vi "MagBoard_n64_Serial_Viewer.vi"() -> ()   [LabVIEW 2018]
uses:
  <vilib>/Math Plots/3D Math Plots/3D Surface/3D Surface XCtrl/3D Surface.xctl
  <vilib>/Utility/file.llb/Write Delimited Spreadsheet (DBL).vi
  <vilib>/Utility/file.llb/Read Delimited Spreadsheet (I64).vi
  <vilib>/Math Plots/3D Math Plots/3D Surface/3D Surface Datatype/Public/Plot Helper (Matrix).vi
  <vilib>/Math Plots/3D Math Plots/3D Surface/3D Surface Datatype/3D Surface Datatype.lvclass
panel:
  out "Reading":bool
  out "Initialised":bool
  out "Connected":bool
  in  "Tab Control":T1(tab)
  out "3D Surface":refnum<class "3D Plot Datatype.lvclass">[](xcontrol)
  out "Node XYZ List":dbl[][](array[numeric])
  in  "dT":u32=40
  in  "Axis":enum16{"X", "Y", "Z", "Calib Z"}(ring)
  out "Real dT":u32
  in  "Tare":bool
  out "Initialisation String":string
  out "Data Packet":string
  out "Time":u32=4294745741
  out "Read Count":i32
  out "Sensor Lookup Indices":i32[](array[numeric])
  in  "VISA resource name":refnum<visa-resource-name>="COM7"
  in  "Serial Settings":T2={"baud rate"=115200, "data bits"=8, "parity"=enum."None", "stop bits"=10, "flow control"=0} {"flow control" items=["None"=0, "XON/XOFF"=1, "RTS/CTS"=2, "DTR/DSR"=4]; "stop bits" items=["1.0"=10, "1.5"=15, "2.0"=20]; "data bits" min=5 max=8 step=1; "baud rate" items=["75"=75, "110"=110, "134"=134, "150"=150, "300"=300, "600"=600, "1200"=1200, "1800"=1800, "2400"=2400, "4800"=4800, "7200"=7200, "9600"=9600, "14400"=14400, "19200"=19200, "28800"=28800, "38400"=38400, "56000"=56000, "57600"=57600, "115200"=115200, "128000"=128000, "230400"=230400]}
  in  "Sensor Lookup_Indices":path=path "C:/Users/menmhou/Documents/Brace+/MagSense/MagBoard_LabVIEW_Client/n64_lookup_file.csv"
  in  "Packet Size (Bytes)":u32=1024
  in  "Gains":dbl[](array[numeric])=[1.502e-06, 1.502e-06, 2.42e-06]
  in  "Export File (CSV)":path=path "C:/Users/menprc/Documents/GitHub/MagLib/MagBoard_n64_UI/MagBoard_n64_UI_LabVIEW_Client/example_data/M064_008.csv"
  in  "Save?":bool
  in  "stop":bool
  # "MagBoard:viewer"
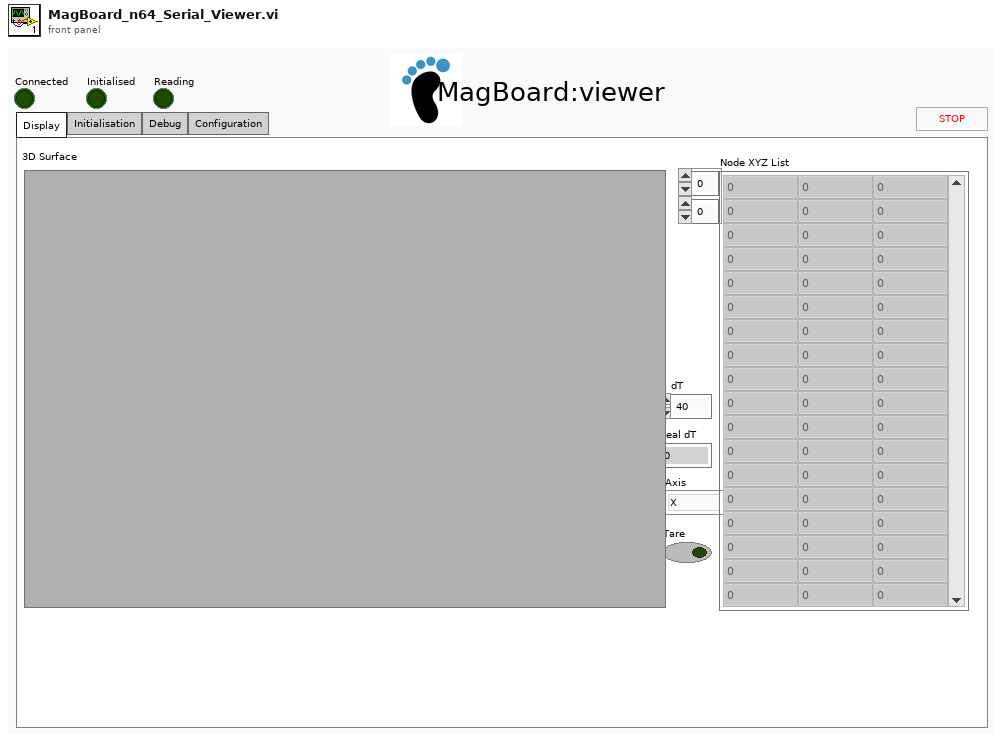
[diagram p1: front panel]
types:
  T1 = enum32{"Display", "Initialisation", "Debug", "Configuration"}
  T2 = cluster{"baud rate":u32, "data bits":u16, "parity":enum16{"None", "Odd", "Even", "Mark", "Space"}, "stop bits":u16, "flow control":u16}
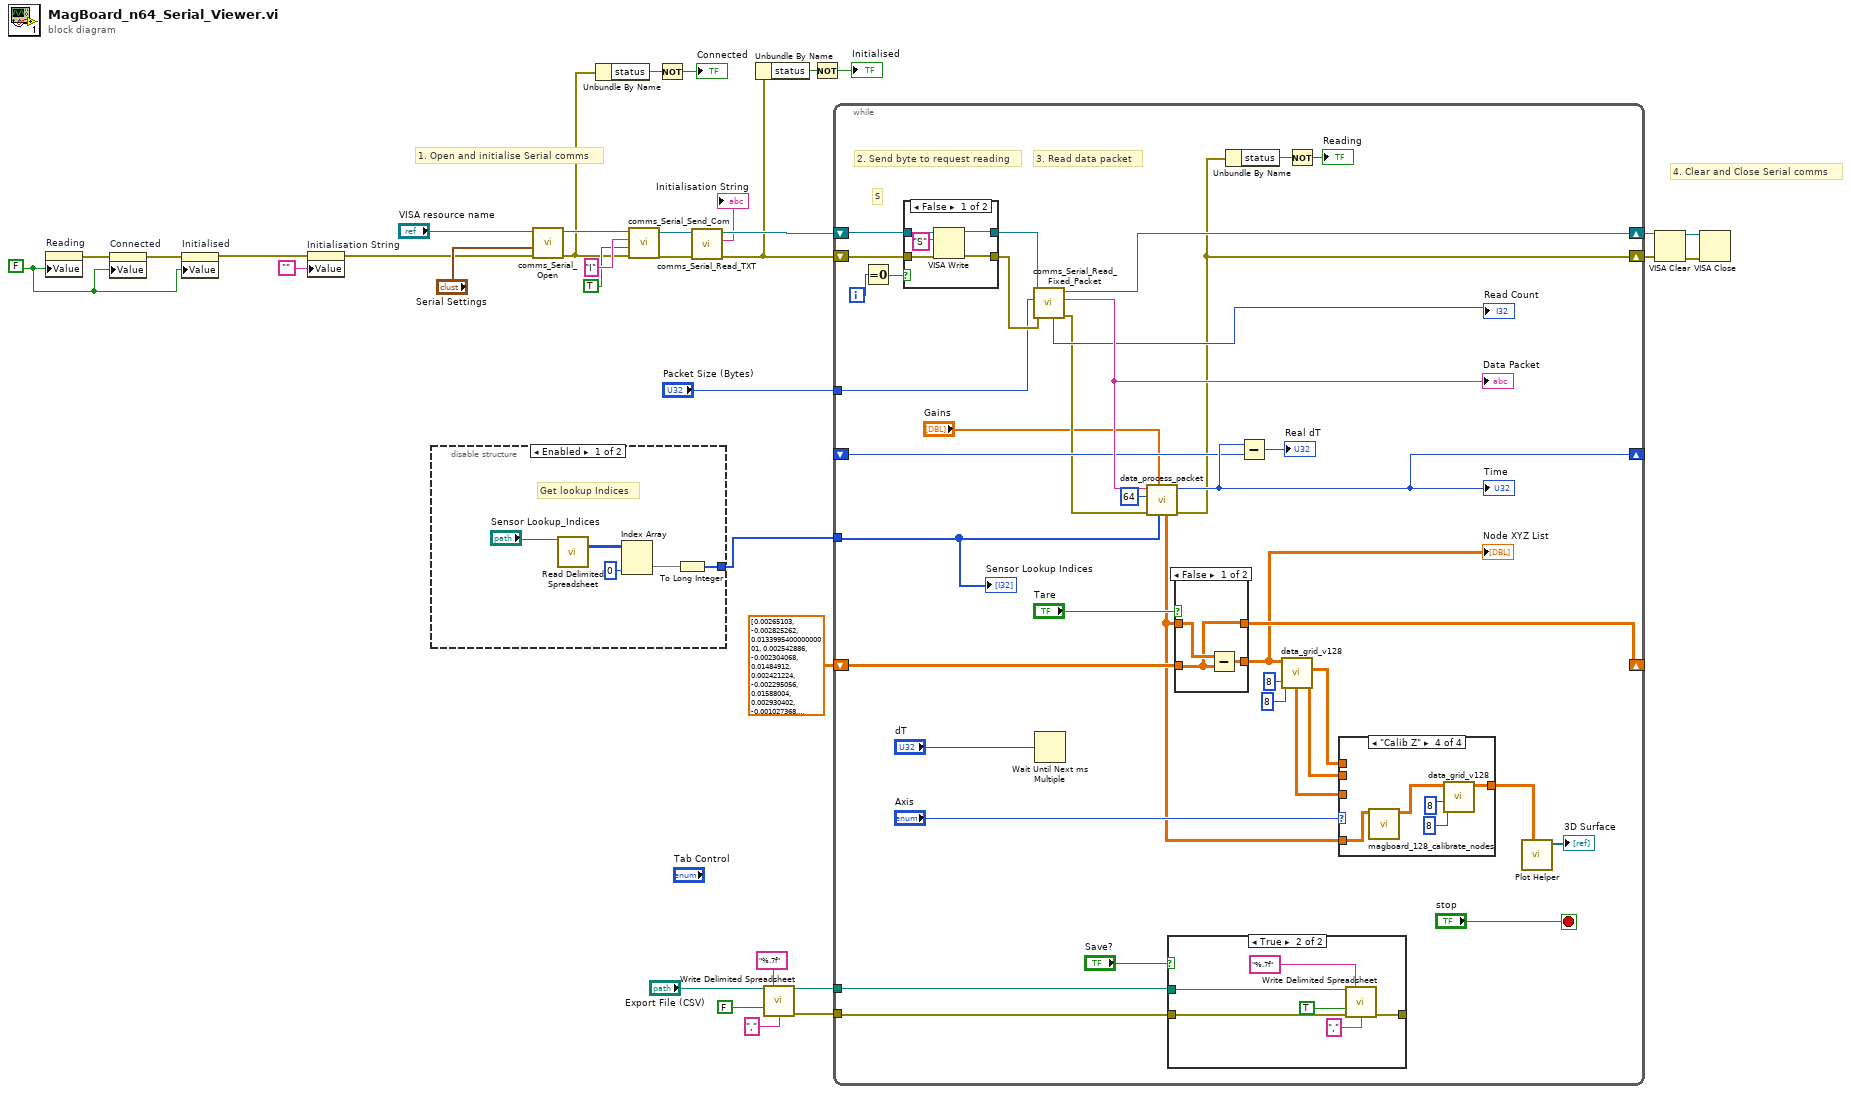
[diagram p0: block diagram]
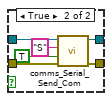
[diagram p5: hidden frame]
diagram:
  w8 = FALSE ("Send Init Comm?")
  # "4. Clear and Close Serial comms"
  # "1. Open and initialise Serial comms"
  n1 = property on="Reading" class="Bool (strict)"("Value"=w8) -> (error out=w10:errorcluster)  [unwired: 2 in, 1 out]
  n2 = property on="Connected" class="Bool (strict)"(error in=w10, "Value"=w8) -> (error out=w11:errorcluster)  [unwired: 1 in, 1 out]
  n3 = property on="Initialised" class="Bool (strict)"(error in=w11, "Value"=w8) -> (error out=w9:errorcluster)  [unwired: 1 in, 1 out]
  n4 = property on="Initialisation String" class="Str"(error in=w9, "Value"="") -> (error out=w32:errorcluster)  [unwired: 1 in, 1 out]
  n5 = disable-structure shown="Enabled" {
    disable-tunnel: [w34 _] -> w1
    frame Enabled {
      # "Get lookup Indices"
      n6 = call-poly <vilib>:"Read Delimited Spreadsheet.vi"("file path (dialog if empty)"="Sensor Lookup_Indices") -> ("all rows"=w37:i64[][])  [unwired: 9 in, 5 out]
      n7 = Index Array(array=w37, index (col)=0 ("disabled index (col)")) -> (element=w35:i64[])  [unwired: 1 in]
      n8 = To Long Integer(number=w35) -> (32bit integer=w34:i32[])
    }
    frame Disabled {
    }
  }
  n9 = call "comms_Serial_Open.vi"("error in (no error)"=w32, "Serial Settings in"="Serial Settings", "VISA Refnum in"="VISA resource name") -> ("error out"=w18:errorcluster, "VISA Refnum out"=w25:refnum<visa-resource-name>)  [unwired: 6 in, 1 out]
  n10 = Unbundle By Name(w18) -> ("status"=w17:bool)
  n11 = call "comms_Serial_Send_Com.vi"("Buffer Clear?"=TRUE, "Command"="I", "VISA resource in"=w25) -> ("VISA resource Out"=w23:refnum<visa-resource-name>)  [unwired: 6 in, 2 out]
  n12 = Not(x=w17) -> (.not. x?=→"Connected":bool)
  n13 = call "comms_Serial_Read_TXT.vi"("error in"=w18, "VISA resource in"=w23) -> ("error out"=w15:errorcluster, "Data Out"=→"Initialisation String":string, "VISA resource Out"=w22:refnum<visa-resource-name>)  [unwired: 6 in, 1 out]
  n14 = Unbundle By Name(w15) -> ("status"=w16:bool)
  n15 = call-poly <vilib>:"Write Delimited Spreadsheet.vi"("file path (dialog if empty)"="Export File (CSV)", "format (%.3f)"="%.7f", "append to file? (new file:F)"=FALSE, "delimiter (\\t)"="," ("delimiter (\\t)")) -> ("new file path (Not A Path if cancelled)"=w3:path, "error out"=w2:errorcluster)  [unwired: 10 in]
  n16 = Not(x=w16) -> (.not. x?=→"Initialised":bool)
  n17 = while {
    shift-right: [w60] -> w28
    shift-left: w22 -> [w71]
    shift-right: [w50] -> w27
    shift-left: w15 -> [w70]
    tunnel: "Packet Size (Bytes)" -> [w58]
    shift-right: [w55] -> _
    shift-left: _ -> [w54]
    shift-right: [w47] -> _
    shift-left: dbl[][] [[0.00265103, -0.002825262, 0.013399540000000001], [0.002542886, -0.002304068, 0.01484912], [0.002421224, -0.002295056, 0.01588004], [0.002930402, -0.001027368, 0.016269660000000002], [0.001703268, -0.001330772, 0.014931400000000001], [0.002885342, 0.00087116, 0.01286956], [0.002412212, 0.001140018, 0.012109680000000001], [0.00304155, 0.002436244, 0.014512740000000001], [0.00335697, -0.002732138, 0.013486660000000001], [0.003328432, -0.001737814, 0.0133705], [0.003393018, -0.0010303719999999999, 0.01234926], [0.002888346, -0.001647694, 0.01545896], [0.00317673, 0.000940252, 0.011957220000000001], [0.002904868, 0.000790052, 0.01184348], [0.003080602, 0.00144192, 0.012100000000000001], [0.002712612, 0.002599962, 0.014292520000000001], [0.004050894, -0.001685244, 0.011277200000000001], [0.003370488, -0.001671726, 0.010919040000000001], [0.003393018, -0.000333444, 0.01085854], [0.003490648, 0.000632342, 0.009798580000000001], [0.00304155, 0.000800566, 0.01086338], [0.003172224, 0.0006804059999999999, 0.01325192], [0.002661544, 0.0007284699999999999, 0.0124267], [0.003917216, 0.0031496939999999998, 0.014265900000000001], [0.00343958, -0.002467786, 0.01067704], [0.003727964, -0.00073598, 0.0095832], [0.0032908819999999997, -0.000865152, 0.01149984], [0.003586776, 1.6522e-05, 0.011872520000000001], [0.00424315, 0.000624832, 0.01268322], [0.0038105739999999997, 0.001891018, 0.0094622], [0.003508672, 0.001688248, 0.009943780000000001], [0.004249158, 0.003272858, 0.011872520000000001], [0.003685908, -0.00205023, 0.010011540000000001], [0.003906702, -0.000223798, 0.00871684], [0.003884172, 0.000166722, 0.00953964], [0.00329689, -9.012e-06, 0.010989220000000001], [0.003040048, 0.00122413, 0.008966100000000001], [0.003885674, 0.0010063399999999999, 0.01206854], [0.002948426, 0.000717956, 0.01158696], [0.002511344, 0.0021028, 0.012211320000000001], [0.00342456, -0.002804234, 0.0119185], [0.004202596, 0.000106642, 0.00901208], [0.003637844, -0.000100634, 0.0092565], [0.003359974, -0.000253838, 0.010827080000000001], [0.00385263, 0.000973296, 0.01177572], [0.003411042, 0.001048396, 0.011616000000000001], [0.003181236, 0.00093124, 0.01289376], [0.004007336, 0.003223292, 0.01344794], [0.004135006, -0.001566586, 0.010367280000000001], [0.003947256, 2.5534e-05, 0.01000912], [0.003873658, 0.000392022, 0.00936782], [0.003753498, 0.000928236, 0.00894674], [0.003654366, 0.001387848, 0.01005994], [0.00299649, 0.001007842, 0.00901208], [0.003167718, 0.000797562, 0.01394162], [0.003806068, 0.003170722, 0.0104423], [0.004749324, -0.00118658, 0.011175560000000001], [0.00395777, 0.000279372, 0.00809006], [0.003758004, 0.0005272019999999999, 0.007964220000000001], [0.004285206, 0.001317254, 0.0093896], [0.003756502, 0.0011955919999999999, 0.01043746], [0.0038150799999999998, 0.0013848439999999999, 0.01262514], [0.00329689, 0.001323262, 0.01245332], [0.00377753, 0.00328187, 0.01108602], [0.004560072, -0.0009657859999999999, 0.00998008], [0.0043603059999999996, 0.0003755, 0.00861278], [0.003798558, 4.0554e-05, 0.00983972], [0.00394275, 0.00070594, 0.00959288], [0.004080934, 0.00118658, 0.0100309], [0.0038616419999999998, 0.00155457, 0.01282842], [0.003755, 0.0018024, 0.01241702], [0.004174058, 0.0034831379999999998, 0.0111804], [0.004346788, -0.001094958, 0.01022934], [0.004516514, 0.000587282, 0.0089903], [0.004542048, 0.000306408, 0.01000912], [0.003555234, 0.000432576, 0.00886204], [0.004124492, 0.001700264, 0.009459780000000001], [0.00353721, 0.001587614, 0.01165472], [0.003983304, 0.00239569, 0.010018800000000001], [0.003733972, 0.003157204, 0.012177440000000001], [0.005712106, 0.000108144, 0.010529420000000001], [0.004794384, 0.000449098, 0.00964854], [0.0052600039999999995, 0.000943256, 0.0116402], [0.004433904, 0.00139686, 0.01077868], [0.003899192, 0.00132927, 0.00872652], [0.004204098, 0.001715284, 0.01258884], [0.0040283639999999996, 0.002093788, 0.01215566], [0.00383761, 0.0031542, 0.01327612], [0.0051113059999999995, -0.00090871, 0.012584000000000001], [0.004342282, 0.00041154799999999997, 0.010360020000000001], [0.004271688, 0.0008351119999999999, 0.00917664], [0.003873658, 0.000459612, 0.011253], [0.003992316, 0.0012676879999999999, 0.01147564], [0.003816582, 0.001829436, 0.00992442], [0.004720786, 0.00313918, 0.011812020000000001], [0.003954766, 0.003564246, 0.01272436], [0.004620152, -0.000579772, 0.01016884], [0.004534538, 0.00015771, 0.01096744], [0.004097456, 0.0008261, 0.009798580000000001], [0.004869484, 0.002078768, 0.009559], [0.00481391, 0.002216952, 0.0111804], [0.0047328019999999995, 0.002284542, 0.011463540000000001], [0.004585606, 0.002526364, 0.01302444], [0.00410797, 0.00382259, 0.010623800000000001], [0.004788376, 0.00051068, 0.00881606], [0.004113978, 0.000687916, 0.00924198], [0.00430323, 0.000919224, 0.008349], [0.0045029959999999996, 0.002002166, 0.00798842], [0.0045811, 0.002347626, 0.01018578], [0.003801562, 0.001988648, 0.009534800000000001], [0.0038601399999999998, 0.00199766, 0.00954206], [0.003849626, 0.00361231, 0.010495540000000001], [0.0053035619999999995, 0.000534712, 0.0102366], [0.004809404, 0.001695758, 0.009365400000000001], [0.004620152, 0.0023446219999999998, 0.006938140000000001], [0.00428821, 0.002239482, 0.00744634], [0.004376828, 0.002604468, 0.0087725], [0.0047823679999999995, 0.003065582, 0.008644240000000001], [0.0041650459999999995, 0.002702098, 0.00852082], [0.003797056, 0.003516182, 0.00851356], [0.005273522, 0.000808076, 0.0105512], [0.005123322, 0.00141939, 0.01190398], [0.005022688, 0.00230557, 0.00889592], [0.004995652, 0.002389682, 0.008908020000000001], [0.004150026, 0.001701766, 0.00965822], [0.0049280619999999995, 0.002389682, 0.01068914], [0.005060238, 0.003179734, 0.01042052], [0.004387342, 0.0036213219999999997, 0.0097889]] ("Node XYZ List") -> [w48]
    tunnel: w3 -> [w44]
    tunnel: w2 -> [w43]
    tunnel: w1 -> [w40]
    i -> [w69]
    stop <- "stop" stop-if-true
    # "3. Read data packet"
    # "2. Send byte to request reading"
    # "S"
    n18 = Equal To 0?(x=w69) -> (x = 0?=w56:bool)
    n19 = case shown="False" w56 {
      tunnel: w71 -> [w92 w98]
      tunnel: w70 -> [w89 w96]
      tunnel: [w91 w95] -> w62
      tunnel: [w88 w94] -> w61
      frame False {
        n20 = VISA Write(VISA resource name=w92, write buffer="S", error in (no error)=w89) -> (VISA resource name out=w91:refnum<visa-resource-name>, error out=w88:errorcluster)  [unwired: 1 out]
      }
      frame True {
        n21 = call "comms_Serial_Send_Com.vi"("error in"=w96, "Buffer Clear?"=TRUE, "Command"="S", "VISA resource in"=w98) -> ("error out"=w94:errorcluster, "VISA resource Out"=w95:refnum<visa-resource-name>)  [unwired: 5 in, 1 out]
      }
    }
    n22 = call "comms_Serial_Read_Fixed_Packet.vi"("error in"=w61, "Packet Size (Bytes)"=w58, "VISA resource in"=w62) -> ("error out"=w52:errorcluster, "Data Out"=w59:string, "VISA resource Out"=w60:refnum<visa-resource-name>, "Bytes Read"=→"Read Count":u32)  [unwired: 4 in, 1 out]
    "Data Packet" <- w59
    n23 = Wait Until Next ms Multiple(millisecond multiple="dT") -> ()  [unwired: 1 out]
    n24 = call "data_process_packet.vi"("Sensor Lookup Indices"=w40, "Gains"="Gains", "error in (no error)"=w52, "No. Sensors"=64 ("No. Nodes"), "Binary Input Data"=w59) -> ("error out"=w50:errorcluster, "Time"=w55:u32, "Sensors (uT)"=w39:dbl[][])  [unwired: 2 in, 2 out]
    "Time" <- w55
    n25 = case shown="True" "Save?" {
      tunnel: w44 -> [_ w80]
      tunnel: w43 -> [w77 w79]
      tunnel: [w77 w78] -> _
      frame False {
      }
      frame True {
        n26 = call-poly <vilib>:"Write Delimited Spreadsheet.vi"("file path (dialog if empty)"=w80, "format (%.3f)"="%.7f", "append to file? (new file:F)"=TRUE, "error in (no error)"=w79, "delimiter (\\t)"="," ("delimiter (\\t)")) -> ("error out"=w78:errorcluster)  [unwired: 9 in, 1 out]
      }
    }
    n27 = case shown="False" "Tare" {
      tunnel: w39 -> [w86 w87]
      tunnel: w48 -> [w84 _]
      tunnel: [w85 w87] -> w45
      tunnel: [w84 w87] -> w47
      frame False {
        n28 = Subtract(x=w86, y=w84) -> (x-y=w85:dbl[][])
      }
      frame True {
      }
    }
    "Node XYZ List" <- w45
    n29 = Unbundle By Name(w50) -> ("status"=w51:bool)
    n30 = Subtract(x=w55, y=w54) -> (x-y=→"Real dT":u32)
    n31 = call "data_grid_v128.vi"("No. Columns"=8, "No. Rows"=8 ("Row Length"), "Sensor Data"=w45) -> ("Y (GRID)"=w65:dbl[][], "X (GRID)"=w66:dbl[][], "Z (GRID)"=w64:dbl[][])  [unwired: 5 in, 1 out]
    n32 = Not(x=w51) -> (.not. x?=→"Reading":bool)
    n33 = case shown="\"Calib Z\"" "Axis" {
      tunnel: w66 -> [w99 _ _ _]
      tunnel: w65 -> [_ w100 _ _]
      tunnel: w64 -> [_ _ w101 _]
      tunnel: [w99 w100 w101 w104] -> w63
      tunnel: w39 -> [_ _ _ w106]
      frame "X", Default {
      }
      frame "Y" {
      }
      frame "Z" {
      }
      frame "Calib Z" {
        n34 = call "magboard_128_calibrate_nodes.vi"("Sensor Input (mT)"=w106) -> ("Sensor Output - Position (mm)"=w103:dbl[][])  [unwired: 10 in]
        n35 = call "data_grid_v128.vi"("No. Columns"=8, "No. Rows"=8 ("Row Length"), "Sensor Data"=w103) -> ("Z (GRID)"=w104:dbl[][])  [unwired: 5 in, 3 out]
      }
    }
    n36 = call-poly <vilib>:"Plot Helper.vi"("z matrix"=w63) -> ("3D Plot lvclass Array out"=→"3D Surface":refnum<class "3D Plot Datatype.lvclass">[])  [unwired: 5 in, 5 out]
    "Sensor Lookup Indices" <- w40
  }
  n37 = VISA Clear(VISA resource name=w28, error in (no error)=w27) -> (VISA resource name out=w30:refnum<visa-resource-name>, error out=w29:errorcluster)
  n38 = VISA Close(VISA resource name=w30, error in (no error)=w29) -> ()  [unwired: 1 out]
